vi "SingleConnection.vi"() -> ()   [LabVIEW 2012]
doc: "This VI acts as a server for an incoming websockets connection. Receives/sends string data to the connected client."
uses:
  WebSockets/WebSockets.lvlib
panel:
  out "Request URI":string
  out "HTTP Headers":variant
  in  "Stop":bool
  out "Received Data":string
  in  "Send":bool
  in  "Data":string
  # "Run this VI and then open the index.html in the package installation directory."
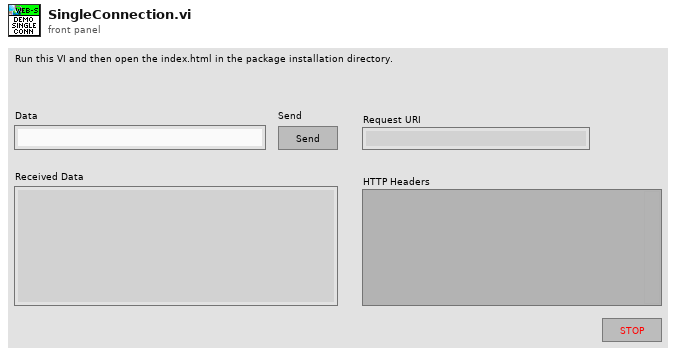
[diagram p1: front panel]
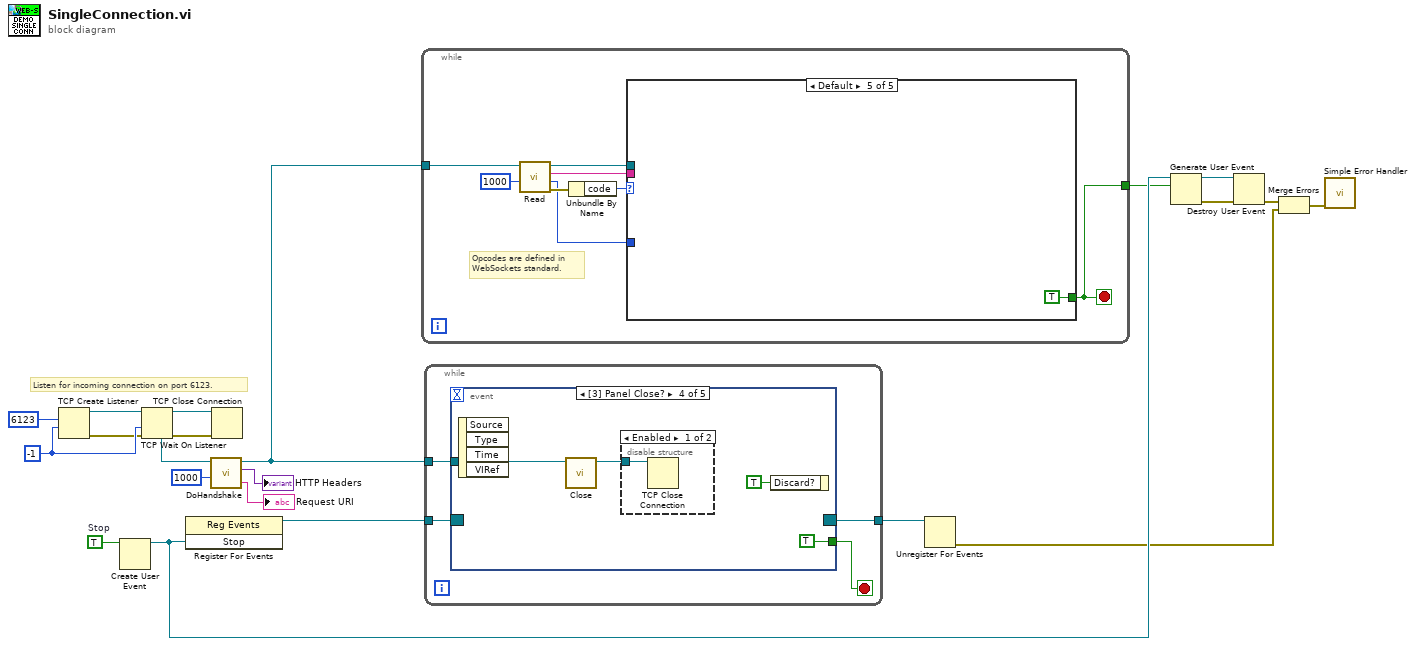
[diagram p0: block diagram]
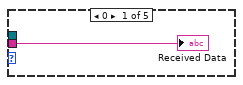
[diagram p2: hidden frame]
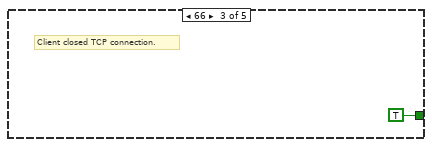
[diagram p4: hidden frame]
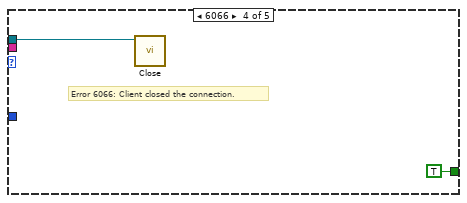
[diagram p5: hidden frame]
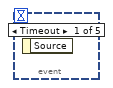
[diagram p6: hidden frame]
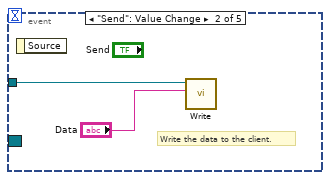
[diagram p7: hidden frame]
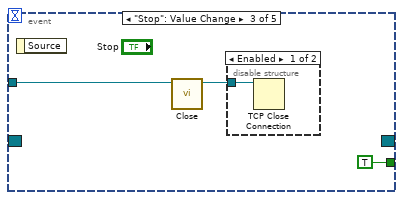
[diagram p8: hidden frame]
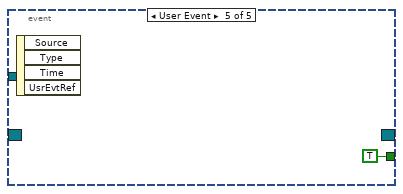
[diagram p11: hidden frame]
diagram:
  w12 = TRUE  # Stop
  w19 = -1 ("timeout ms (25000)")
  # "Listen for incoming connection on port 6123."
  n1 = TCP Create Listener(9:w19, 10:u16 6123 ("port")) -> (0:w17:errorcluster, 3:w18:refnum<k5>)  [unwired: 3 in, 1 out]
  n2 = Create User Event(user event datatype=w12) -> (user event=w10:refnum<user-event>)  [unwired: 1 in, 1 out]
  n3 = TCP Wait On Listener(8:w17, 9:w19, 11:w18) -> (0:w14:errorcluster, 3:w15:refnum<k5>, 4:w16:refnum<k5>)  [unwired: 1 in, 2 out]
  n4 = register-events(w10) -> (reference out=w13:refnum<event-registration>)  [unwired: 2 in, 1 out]
  n5 = call "DoHandshake.vi"("timeout ms (5000)"=1000 ("timeout ms (25000)"), "WebSocket Connection in"=w16) -> ("Request URI"=→"Request URI":string, "Headers Out"=→"HTTP Headers":variant, "WebSocket Connection out"=w21:refnum<k5>)  [unwired: 6 in, 1 out]
  n6 = TCP Close Connection(connection ID=w15, error in (no error)=w14) -> ()  [unwired: 1 in, 2 out]
  n7 = while {
    tunnel: w21 -> [w29]
    tunnel: [w24] -> w9
    stop <- w24 stop-if-true
    # "Opcodes are defined in\nWebSockets standard."
    n8 = call "Read.vi"("timeout ms (5000)"=1000 ("timeout ms (25000)"), "WebSocket Connection in"=w29) -> ("error out"=w27:errorcluster, "Opcode"=w22:u8, "Data"=w25:string, "WebSocket Connection out"=w23:refnum<k5>)  [unwired: 6 in]
    n9 = Unbundle By Name(w27) -> ("code"=w26:i32)
    n10 = case shown="Default" w26 {
      tunnel: w25 -> [w30 _ _ _ _]
      tunnel: [_ _ TRUE TRUE TRUE] -> w24
      tunnel: w23 -> [_ _ _ w33 _]
      tunnel: w22 -> [_ _ _ _ _]
      frame 0 {
        "Received Data" <- w30
      }
      frame 56 {
        # "Read VI timed out."
      }
      frame 66 {
        # "Client closed TCP connection."
      }
      frame 6066 {
        # "Error 6066: Client closed the connection."
        n11 = call "Close.vi"("WebSocket Connection in"=w33) -> ()  [unwired: 9 in, 2 out]
      }
      frame Default {
      }
    }
  }
  n12 = while {
    tunnel: w21 -> [w38]
    tunnel: w13 -> [w36]
    tunnel: [w35] -> w11
    stop <- w37 stop-if-true
    n13 = event shown="[3] Panel Close?" {
      selector: w36 -> [_ _ _ _ _]
      dyn-events: [_ _ _ _ _] -> w35
      timeout: _ -> [_ _ _ _ _]
      tunnel: w38 -> [_ w40 w42 w47 _]
      tunnel: [_ _ TRUE TRUE TRUE] -> w37
      event Timeout {
        n14 = event-data() -> ()  [unwired: 1 in, 1 out]
      }
      event "Send": Value Change {
        # "Write the data to the client."
        n15 = event-data() -> ()  [unwired: 1 in, 1 out]
        n16 = call "Write.vi"("Data"="Data", "WebSocket Connection in"=w40) -> ()  [unwired: 8 in, 2 out]
      }
      event "Stop": Value Change {
        n17 = event-data() -> ()  [unwired: 1 in, 1 out]
        n18 = call "Close.vi"("WebSocket Connection in"=w42) -> ("WebSocket Connection in"=w41:refnum<k5>)  [unwired: 9 in, 1 out]
        n19 = disable-structure shown="Enabled" {
          disable-tunnel: w41 -> [w44 _]
          frame Enabled {
            n20 = TCP Close Connection(connection ID=w44) -> ()  [unwired: 2 in, 2 out]
          }
          frame Disabled {
          }
        }
      }
      event Panel Close? {
        n21 = event-data() -> ()  [unwired: 1 in, 4 out]
        n22 = call "Close.vi"("WebSocket Connection in"=w47) -> ("WebSocket Connection in"=w46:refnum<k5>)  [unwired: 9 in, 1 out]
        n23 = disable-structure shown="Enabled" {
          disable-tunnel: w46 -> [w49 _]
          frame Enabled {
            n24 = TCP Close Connection(connection ID=w49) -> ()  [unwired: 2 in, 2 out]
          }
          frame Disabled {
          }
        }
        n25 = event-data("Discard?"=TRUE) -> ()  [unwired: 1 in, 1 out]
      }
      event User Event {
        n26 = event-data() -> ()  [unwired: 1 in, 4 out]
      }
    }
  }
  n27 = Unregister For Events(event registration refnum=w11) -> (error out=w5:errorcluster)  [unwired: 1 in]
  n28 = Generate User Event(user event=w10, event data cluster=w9) -> (user event out=w8:refnum<user-event>, error out=w7:errorcluster)  [unwired: 1 in]
  n29 = Destroy User Event(user event=w8, error in=w7) -> (error out=w6:errorcluster)
  n30 = Merge Errors(w6, w5) -> (w1:errorcluster)
  n31 = call <vilib>:"Simple Error Handler.vi"("error in (no error)"=w1) -> ()  [unwired: 4 in, 5 out]
